vi "OpenDevice.vi"(10 "Waveform Specification":T1={"X SignalType"=enum."Sine Wave", "X Offset"=2.0, "X Frequency"=100.0, "X Amplitude"=1.0, "X Phase"=0.0, "Y SignalType"=enum."Sine Wave", "Y Offset"=2.0, "Y Frequency"=100.0, "Y Amplitude"=1.0, "Y Phase"=0.0, "Z SignalType"=enum."Sine Wave", "Z Offset"=2.0, "Z Frequency"=100.0, "Z Amplitude"=1.0, "Z Phase"=0.0}) -> (0 "error out":errorcluster, 2 "Array":waveform(dbl)[](array[waveform]), 3 "Refnum out":refnum<k21>)   [LabVIEW 2017, in "WaveformGenerator.lvlib"]
uses:
  WaveformGenerator.lvlib
  WaveformSpecs.ctl
  <vilib>/DAQmx/write.llb/DAQmx Write (Analog 1D Wfm NChan NSamp).vi
  <vilib>/DAQmx/configure/timing.llb/DAQmx Timing (Sample Clock).vi
  <vilib>/DAQmx/miscellaneous.llb/DAQmx Fill In Error Info.vi
  <resource>/objmgr/daqmx.rc
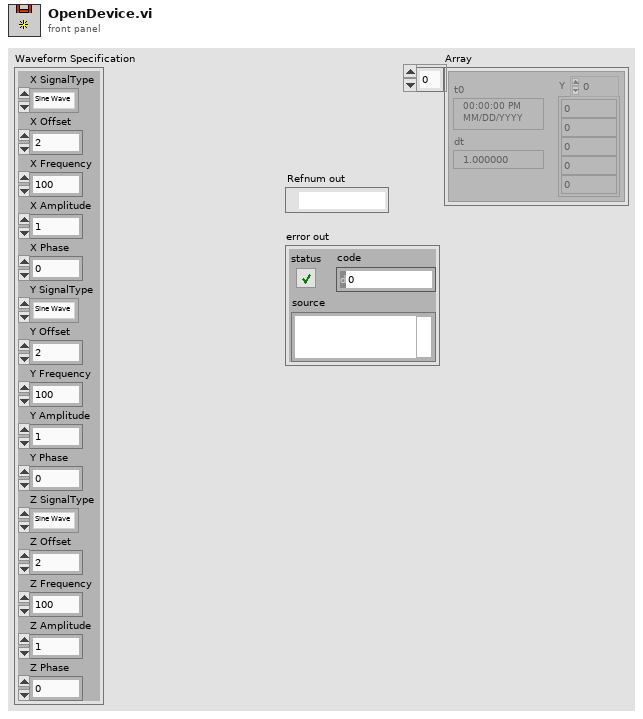
[diagram p1: front panel]
types:
  T1 = typedef "WaveformGenerator.lvlib/WaveformSpecs.ctl" = cluster{"X SignalType":enum16{"Sine Wave", "Triangle Wave", "Square Wave", "Sawtooth Wave"}, "X Offset":dbl, "X Frequency":dbl, "X Amplitude":dbl, "X Phase":dbl, "Y SignalType":enum16{"Sine Wave", "Triangle Wave", "Square Wave", "Sawtooth Wave"}, "Y Offset":dbl, "Y Frequency":dbl, "Y Amplitude":dbl, "Y Phase":dbl, "Z SignalType":enum16{"Sine Wave", "Triangle Wave", "Square Wave", "Sawtooth Wave"}, "Z Offset":dbl, "Z Frequency":dbl, "Z Amplitude":dbl, "Z Phase":dbl}
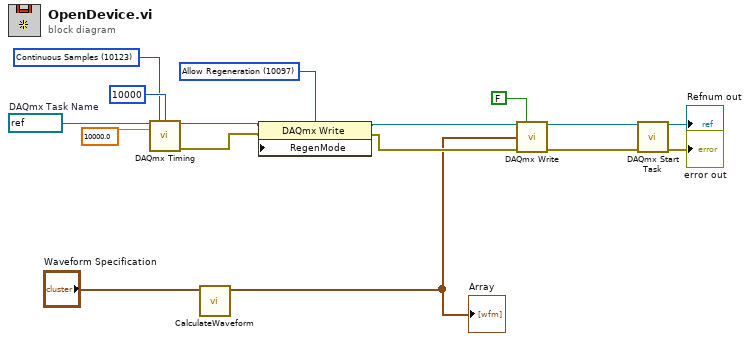
[diagram p0: block diagram]
diagram:
  w16 = 10097 items=["Allow Regeneration"=10097, "Do Not Allow Regeneration"=10158] ("RegenMode")
  w11 = 10123 items=["Finite Samples"=10178, "Continuous Samples"=10123, "Hardware Timed Single Point"=12522] ("sample mode")
  w10 = refnum<k21> "Coils"  # DAQmx Task Name
  n1 = call-poly <vilib>:"DAQmx Timing.vi"("task/channels in"=w10, "sample mode"=w11, "samples per channel"=10000, "rate"=10000.0) -> ("task out"=w14:refnum<k21>, "error out"=w15:errorcluster)  [unwired: 10 in]
  n2 = call "CalculateWaveform.vi"("Waveform Specification"="Waveform Specification") -> ("Array"=w1:waveform(dbl)[])  [unwired: 9 in, 1 out]
  "Array" <- w1
  n3 = property class="DAQmx Write"(reference=w14, error in=w15, "RegenMode"=w16) -> (reference out=w3:refnum<k21>, error out=w5:errorcluster)
  n4 = call-poly <vilib>:"DAQmx Write.vi"("task/channels in"=w3, "auto start"=FALSE, "data"=w1, "error in"=w5) -> ("task out"=w4:refnum<k21>, "error out"=w6:errorcluster)  [unwired: 9 in, 1 out]
  n5 = call <vilib>:"DAQmx Start Task.vi"("task/channels in"=w4, "error in"=w6) -> ("task out"=→"Refnum out":refnum<k21>, "error out"=→"error out":errorcluster)  [unwired: 12 in]
